vi "Message_OnlyShow.vi"(8 "error in (no error)":errorcluster caption="错误输入（无错误）", 10 "信息":string, 11 "引用":string) -> (0 "error out":errorcluster caption="错误输出", 3 "引用":string)   [LabVIEW 2012, in "Message.lvlib"]
uses:
  Message.lvlib
  Message.ctl
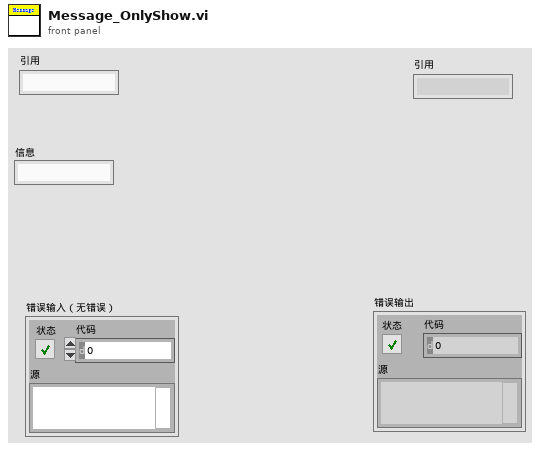
[diagram p1: front panel]
types:
  T1 = typedef "Message.lvlib/Message.ctl" = cluster{"LogPath":path, "信息框引用":refnum<vi>}
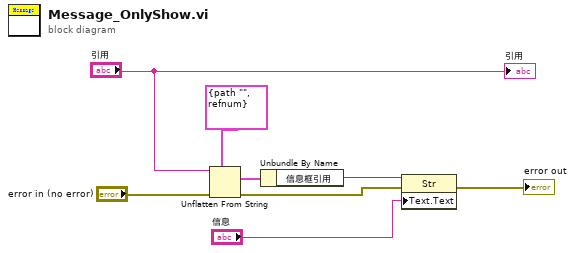
[diagram p0: block diagram]
diagram:
  n1 = Unflatten From String(type=T1 {"LogPath"=path "", "信息框引用"=refnum} ("文本显示引用"), binary string="引用", error in (no error)="error in (no error)") -> (value=w6:T1, error out=w4:errorcluster)  [unwired: 2 in, 1 out]
  n2 = Unbundle By Name(w6) -> ("信息框引用"=w5:refnum<vi>)
  n3 = property class="Str"(reference=w5, error in=w4, "Text.Text"="信息") -> (error out=→"error out":errorcluster)  [unwired: 1 out]
  "引用" <- "引用"
